vi "Operaciones_Senales.vi"() -> ()   [LabVIEW 2016]
uses:
  <vilib>/DAQmx/read.llb/DAQmx Read (Analog 1D DBL 1Chan NSamp).vi
  <vilib>/DAQmx/create/channels.llb/DAQmx Create Channel (AI-Voltage-Basic).vi
  <vilib>/DAQmx/configure/timing.llb/DAQmx Timing (Sample Clock).vi
  <vilib>/DAQmx/miscellaneous.llb/DAQmx Fill In Error Info.vi
  <vilib>/imath/engines/lvmath2/RunTimeEngine/BuiltInFunctions/length/NIMS_length(GV).vi
  <instcachedir>/0/NIMS_length(GV)_08A3D13377FD4E4B96F5795FBF3698FA.lvgen/NIMS_length(GV)_08A3D13377FD4E4B96F5795FBF3698FA_000.vi
  <vilib>/imath/engines/lvmath2/RunTimeEngine/RangeToken/NIMS_Range.vi
  <instcachedir>/0/NIMS_Range_A7C094595B484CA7AF10685B02D808ED.lvgen/NIMS_Range_A7C094595B484CA7AF10685B02D808ED_001.vi
  <vilib>/imathl/engines/lvmath/Functions/Error Handling/Create Error.vi
  <vilib>/imath/engines/lvmath2/RunTimeEngine/IndexReplace/NIMS V(S)=S.vi
  <instcachedir>/0/NIMS V(S)=S_57E16554CB8B4B90AAB163894F717546.lvgen/NIMS V(S)=S_57E16554CB8B4B90AAB163894F717546_003.vi
  <vilib>/imath/engines/lvmath2/RunTimeEngine/RangeToken/NIMS_Range_R2 - Integer.vi
  <instcachedir>/0/NIMS_Range_R2 - Integer_89B873E74E6E489885E44F751DD9C6BF.lvgen/NIMS_Range_R2 - Integer_89B873E74E6E489885E44F751DD9C6BF_000.vi
  <vilib>/imath/engines/lvmath2/RunTimeEngine/CommandStatement/MC_CommandStatement_break.vi
  <vilib>/imath/engines/lvmath2/RunTimeEngine/IndexRead/NIMS V(S).vi
  <instcachedir>/0/NIMS V(S)_0488751826AF41519A22953C041130DC.lvgen/NIMS V(S)_0488751826AF41519A22953C041130DC_000.vi
  <instcachedir>/0/NIMS V(S)=S_57E16554CB8B4B90AAB163894F717546.lvgen/NIMS V(S)=S_57E16554CB8B4B90AAB163894F717546_000.vi
  <vilib>/imath/engines/lvmath2/RunTimeEngine/ErrorHandling/NIMS_Create Error From Enums.vi
  <vilib>/imath/engines/lvmath2/RunTimeEngine/NodeEndStatement/NIMS_NodeEndStatement_Output.vi
  <instcachedir>/0/NIMS_NodeEndStatement_Output_53EC0D466D134D7ABD903AC30B43404B.lvgen/NIMS_NodeEndStatement_Output_53EC0D466D134D7ABD903AC30B43404B_005.vi
  <vilib>/imath/engines/lvmath2/RunTimeEngine/ErrorHandling/NIMS_Finalize Error.vi
panel:
  out "Integral":cluster{"Tiempo":dbl[], "Entrada":dbl[]}(graph)
  out "Derivada":cluster{"Tiempo":dbl[], "Entrada":dbl[]}(graph)
  out "Entrada":cluster{"Tiempo":dbl[], "Entrada":dbl[]}(graph)
  out "data":dbl[](graph)
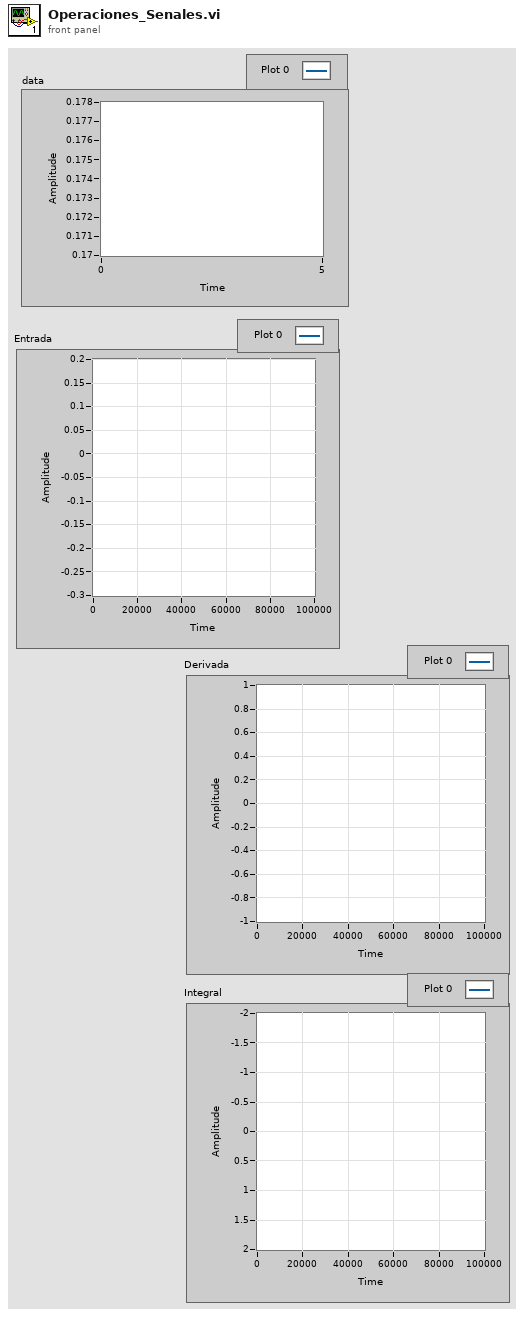
[diagram p1: front panel]
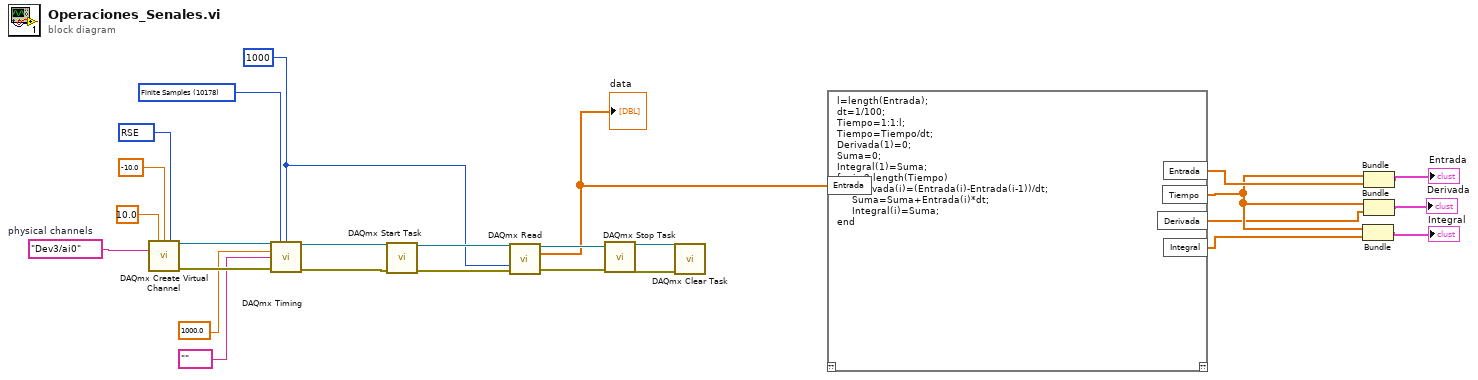
[diagram p0: block diagram]
diagram:
  w13 = 1000 ("samples per channel")
  w22 = 10178 items=["Finite Samples"=10178, "Continuous Samples"=10123, "Hardware Timed Single Point"=12522] ("sample mode")
  w23 = tag "Dev3/ai0"  # physical channels
  w26 = 10083 items=["Default"=-1, "RSE"=10083, "NRSE"=10078, "Differential"=10106, "Pseudodifferential"=12529] ("input terminal configuration")
  n1 = call-poly <vilib>:"DAQmx Create Virtual Channel.vi"("maximum value"=10.0, "minimum value"=-10.0, "input terminal configuration"=w26, "physical channels"=w23) -> ("task out"=w21:refnum<k21>, "error out"=w20:errorcluster)  [unwired: 10 in]
  n2 = call-poly <vilib>:"DAQmx Timing.vi"("task/channels in"=w21, "sample mode"=w22, "samples per channel"=w13, "rate"=1000.0, "source"=tag "", "error in"=w20) -> ("task out"=w17:refnum<k21>, "error out"=w15:errorcluster)  [unwired: 8 in]
  n3 = call <vilib>:"DAQmx Start Task.vi"("task/channels in"=w17, "error in"=w15) -> ("task out"=w16:refnum<k21>, "error out"=w14:errorcluster)  [unwired: 12 in]
  n4 = call-poly <vilib>:"DAQmx Read.vi"("task/channels in"=w16, "timeout"=w13, "error in"=w14) -> ("task out"=w11:refnum<k21>, "data"=w8:dbl[], "error out"=w12:errorcluster)  [unwired: 10 in]
  "data" <- w8
  n5 = call <vilib>:"DAQmx Stop Task.vi"("task/channels in"=w11, "error in"=w12) -> ("task out"=w10:refnum<k21>, "error out"=w9:errorcluster)  [unwired: 12 in]
  n6 = call <vilib>:"DAQmx Clear Task.vi"("task in"=w10, "error in"=w9) -> ()  [unwired: 13 in, 1 out]
  n7 = mathscript code="l=length(Entrada);\ndt=1/100;\nTiempo=1:1:l;\nTiempo=Tiempo/dt;\nDerivada(1)=0;\nSuma=0;\nIntegral(1)=Suma;\nfor i=2:length(Tiempo)\n     Derivada(i)=(Entrada(i)-Entrada(i-1))/dt;\n     Suma=Suma+Entrada(i)*dt;\n     Integral(i)=Suma;\nend"("Entrada"=w8) -> ("Entrada"=w7:dbl[], "Tiempo"=w6:dbl[], "Derivada"=w5:dbl[], "Integral"=w4:dbl[])  [unwired: 1 in, 1 out]
  n8 = Bundle("Tiempo"=w6, "Integral"=w4) -> (→"Integral":cluster{"Tiempo":dbl[], "Integral":dbl[]})  [unwired: 1 in]
  n9 = Bundle("Tiempo"=w6, "Entrada"=w7) -> (→"Entrada":cluster{"Tiempo":dbl[], "Entrada":dbl[]})  [unwired: 1 in]
  n10 = Bundle("Tiempo"=w6, "Derivada"=w5) -> (→"Derivada":cluster{"Tiempo":dbl[], "Derivada":dbl[]})  [unwired: 1 in]
